vi "Generate Status Line.vi"(11 "状态码":u16) -> (3 "状态行":string)   [LabVIEW 2019, in "HTTP Server.lvlib"]
uses:
  HTTP Server.lvlib
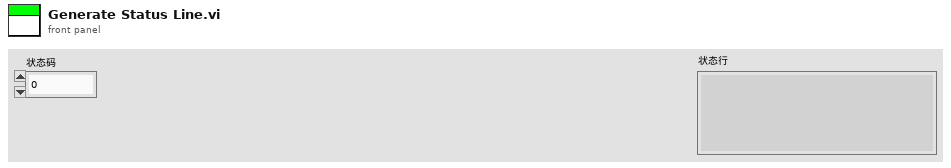
[diagram p1: front panel]
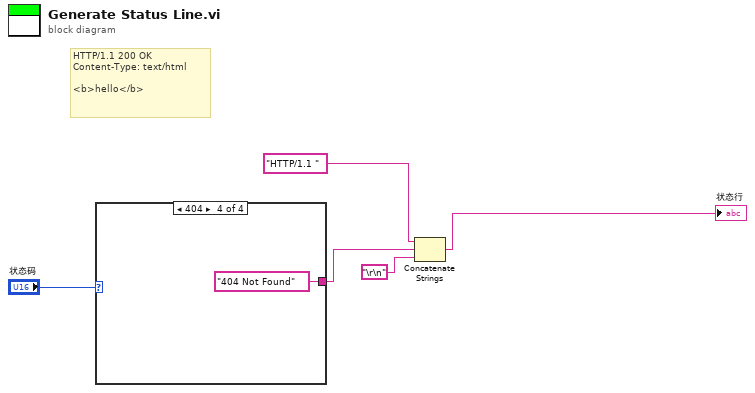
[diagram p0: block diagram]
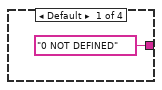
[diagram p2: hidden frame]
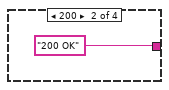
[diagram p3: hidden frame]
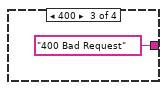
[diagram p4: hidden frame]
diagram:
  # "HTTP/1.1 200 OK\nContent-Type: text/html\n\n<b>hello</b>"
  n1 = case shown="404" "状态码" {
    tunnel: ["0 NOT DEFINED" "200 OK" "400 Bad Request" "404 Not Found"] -> w3
    frame Default {
    }
    frame 200 {
    }
    frame 400 {
    }
    frame 404 {
    }
  }
  n2 = Concatenate Strings("HTTP/1.1 ", w3, "\r\n") -> (→"状态行":string)
